vi "Write bitfile path.vi"(8 "error in (no error)":errorcluster, 10 "bitfile path":path, 11 "FPGA Device in":refnum<class "FPGA Device.lvclass">) -> (0 "error out":errorcluster, 3 "FPGA Device out":refnum<class "FPGA Device.lvclass">)   [LabVIEW 2016, in "FPGA RM Shared API.lvlib" / "FPGA Device.lvclass"]
uses:
  FPGA Device.lvclass
  FPGA Device.lvclass/FPGA Device.ctl
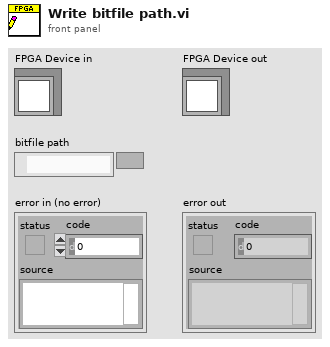
[diagram p1: front panel]
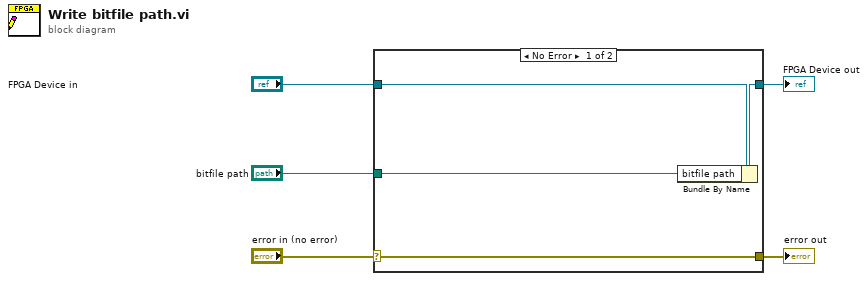
[diagram p0: block diagram]
diagram:
  n1 = case shown="No Error" "error in (no error)" {
    selector: "error in (no error)" -> [w9 w10]
    tunnel: [w9 w10] -> w4
    tunnel: [w7 w11] -> w2
    tunnel: "FPGA Device in" -> [w8 w11]
    tunnel: "bitfile path" -> [w6 _]
    frame No Error {
      n2 = Bundle By Name(cluster=w8, "bitfile path"=w6) -> (w7:refnum<class "FPGA Device.lvclass">)
    }
    frame Error {
    }
  }
  "error out" <- w4
  "FPGA Device out" <- w2
